vi "Query.vi"(8 "error in (no error)":errorcluster, 10 "Query":u16(ring) items=["Measurement Items", "Measurement Values", "Blanking Setting", "Calibration Date", "Frequency Source", "Product ID", "Operating Mode", "Voltage Range", "Current Range", "Voltage Scaling Factor", "Current Scaling Factor", "Shunt Setting", "Auto Zero Setting"], 11 "VISA resource name":refnum<visa-resource-name>) -> (0 "error out":errorcluster, 2 "Result":string, 3 "VISA resource name out":refnum<visa-resource-name>)   [LabVIEW 2015, in "Voltech PM1000+.lvlib"]
doc: "Queries information from instrument."
uses:
  <instrlib>/Voltech PM1000+/Voltech PM1000+.lvlib
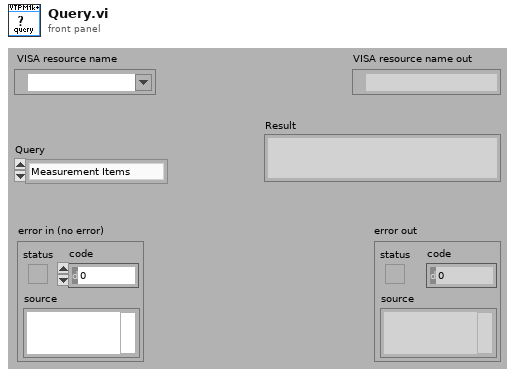
[diagram p1: front panel]
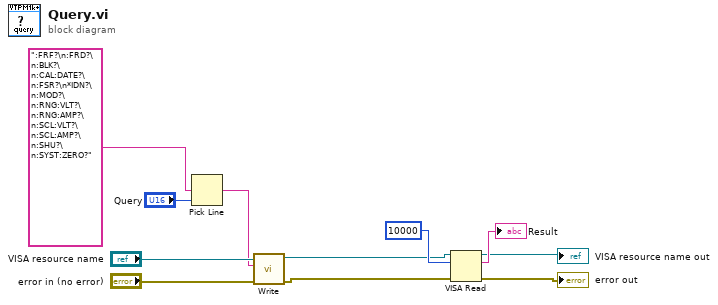
[diagram p0: block diagram]
diagram:
  n1 = Pick Line(multi-line string=":FRF?\n:FRD?\n:BLK?\n:CAL:DATE?\n:FSR?\n*IDN?\n:MOD?\n:RNG:VLT?\n:RNG:AMP?\n:SCL:VLT?\n:SCL:AMP?\n:SHU?\n:SYST:ZERO?", line index="Query") -> (output string=w5:string)  [unwired: 1 in]
  n2 = call <instrlib>:"Write.vi"("error in (no error)"="error in (no error)", "Write Buffer"=w5, "VISA resource name"="VISA resource name") -> ("error out"=w3:errorcluster, "VISA resource name out"=w4:refnum<visa-resource-name>)  [unwired: 7 in]
  n3 = VISA Read(VISA resource name=w4, byte count=u32 10000, error in (no error)=w3) -> (VISA resource name out=→"VISA resource name out":refnum<visa-resource-name>, read buffer=→"Result":string, error out=→"error out":errorcluster)  [unwired: 1 out]
